vi "Obtain Byte Buffer.vi"(8 "error in (no error)":errorcluster, 11 "Transfer Runtime in":refnum<class "Runtime.Transfer.lvclass">) -> (0 "error out":errorcluster, 2 "Byte Buffer":refnum<class "Byte Buffer.lvclass">, 3 "Transfer Runtime out":refnum<class "Runtime.Transfer.lvclass">)   [LabVIEW 2016, in "Data Sharing Framework.Runtime.lvlib" / "Runtime.Transfer.lvclass"]
uses:
  Runtime.Transfer.lvclass
  <vilib>/NI Veristand/VeriStand Data/Byte Buffer/Byte Buffer.lvclass
  Runtime.Transfer.lvclass/Runtime.Transfer.ctl
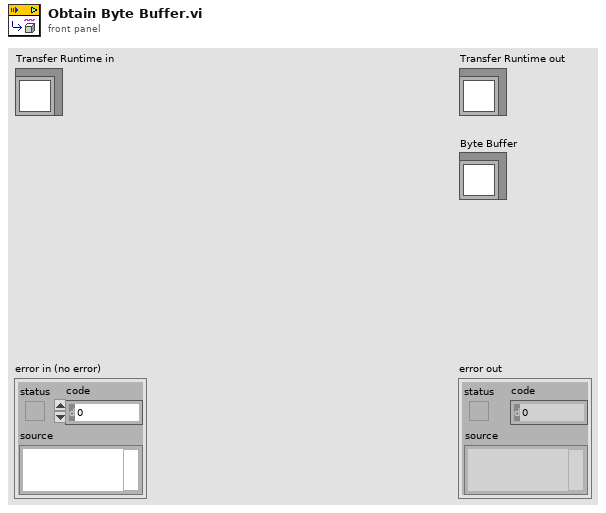
[diagram p1: front panel]
types:
  T1 = enum16{"big-endian, network order", "native, host order", "little-endian"}
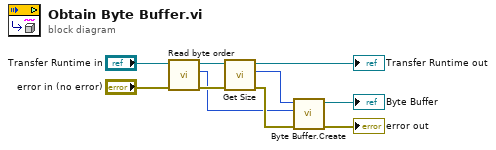
[diagram p0: block diagram]
diagram:
  n1 = call "Read byte order.vi"("error in (no error)"="error in (no error)", "Runtime.Transfer in"="Transfer Runtime in") -> ("error out"=w7:errorcluster, "byte order"=w4:T1, "Runtime.Transfer out"=w8:refnum<class "Runtime.Transfer.lvclass">)  [unwired: 7 in]
  n2 = call "Get Size.vi"("error in (no error)"=w7, "Transfer Runtime in"=w8) -> ("error out"=w5:errorcluster, "size in bytes"=w3:u64, "Transfer Runtime out"=→"Transfer Runtime out":refnum<class "Runtime.Transfer.lvclass">)  [unwired: 7 in]
  n3 = call <vilib>:"Byte Buffer.Create.vi"("error in (no error)"=w5, "byte order (big-endian)"=w4, "size"=w3) -> ("error out"=→"error out":errorcluster, "Byte Buffer"=→"Byte Buffer":refnum<class "Byte Buffer.lvclass">)  [unwired: 7 in]
